vi "Reset stages speed.vi"(8 "error in (no error)":errorcluster, 11 "Tomo in":refnum<class "Invivo_Tomo.lvclass">) -> (0 "error out":errorcluster, 3 "Tomo out":refnum<class "Invivo_Tomo.lvclass">)   [LabVIEW 2012, in "Invivo_Tomo.lvclass"]
uses:
  Invivo_Tomo.lvclass
  <vilib>/Distrio/Murmex/Murmex/update_cluster.ctl
  Invivo_Tomo.lvclass/Invivo_Tomo.ctl
  <vilib>/Distrio/Murmex/Murmex/Murmex.lvclass
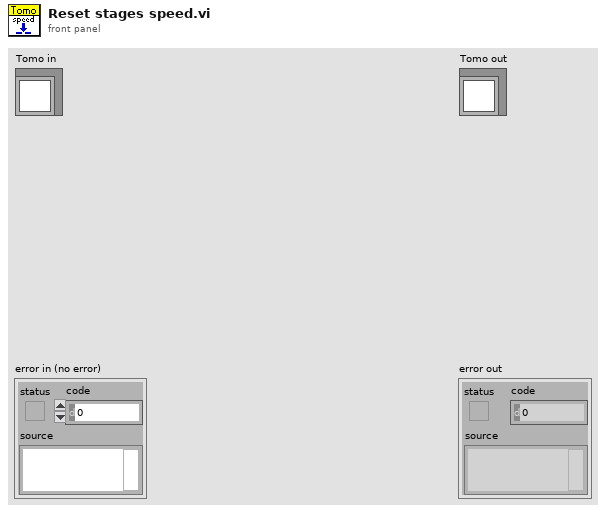
[diagram p1: front panel]
types:
  T1 = typedef "Murmex.lvlib/Murmex.lvclass/update_cluster.ctl" = cluster{"target ID":string, "key chains":string[], "values":variant[]}
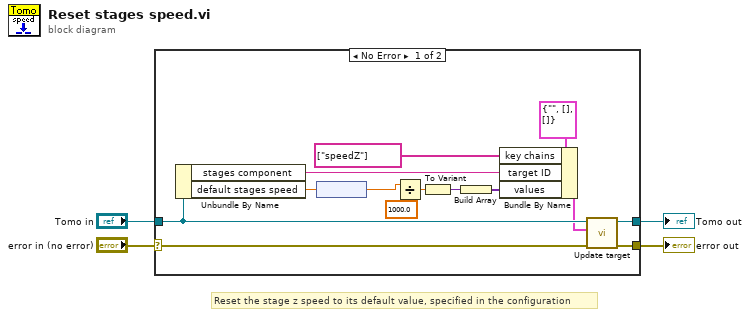
[diagram p0: block diagram]
diagram:
  # "Reset the stage z speed to its default value, specified in the configuration"
  n1 = case shown="No Error" "error in (no error)" {
    selector: "error in (no error)" -> [w17 w20]
    tunnel: [w16 w20] -> w3
    tunnel: [w14 w19] -> w1
    tunnel: "Tomo in" -> [w15 w19]
    frame No Error {
      n2 = Unbundle By Name(w15) -> ("stages component"=w10:string, "default stages speed"=w13:dbl[unit])
      n3 = node(w13) -> (w6:dbl)
      n4 = Divide(x=w6, y=1000.0) -> (x/y=w5:dbl)
      n5 = To Variant(anything=w5) -> (Variant=w12:variant)
      n6 = Build Array(w12) -> (w11:variant[])
      n7 = Bundle By Name(cluster=T1 {"target ID"="", "key chains"=[], "values"=[]} ("update cluster"), "key chains"=string[] ["speedZ"], "target ID"=w10, "values"=w11) -> (w8:T1)
      n8 = call <vilib>:"Update target.vi"("error in (no error)"=w17, "update cluster"=w8, "MurmexBase in"=w15) -> ("error out"=w16:errorcluster, "MurmexBase out"=w14:refnum<class "Invivo_Tomo.lvclass">)  [unwired: 7 in]
    }
    frame Error {
    }
  }
  "error out" <- w3
  "Tomo out" <- w1
